vi "subLoadCommandlineArgs.vi"(11 "Options in":T4={"Path"=path "C:/DependencyInspector/src", "Preview?"=FALSE, "Quiet?"=FALSE, "Show help?"=FALSE}) -> (0 "error out":errorcluster, 1 "From command line?":bool, 2 "Item info":T1, 3 "Options":T4={"Path"=path "C:/DependencyInspector/src", "Preview?"=FALSE, "Quiet?"=FALSE, "Show help?"=FALSE})   [LabVIEW 2020, in "SolutionBuilder.lvlib" / "SolutionBuilder.lvclass"]
uses:
  SolutionBuilder.lvclass
  Private/Options.ctl
  Private/FileInfo.ctl
  Private/ProjectInfo.ctl
  Private/ItemInfo.ctl
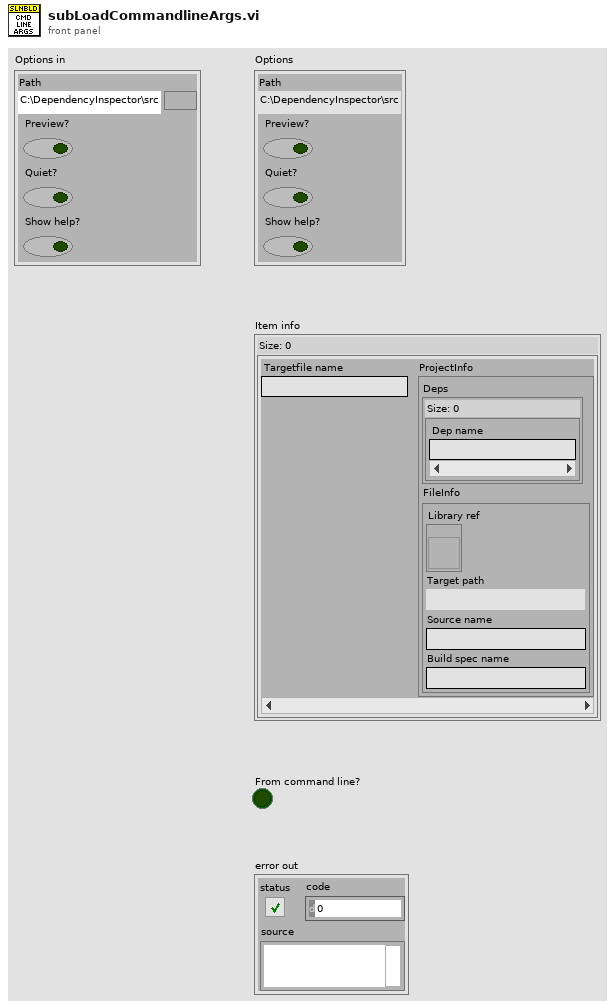
[diagram p1: front panel]
types:
  T1 = typedef "SolutionBuilder.lvlib/SolutionBuilder.lvclass/ItemInfo.ctl" = map{string, T2}
  T2 = typedef "SolutionBuilder.lvlib/SolutionBuilder.lvclass/ProjectInfo.ctl" = cluster{"Deps":set{string}, "FileInfo":T3}
  T3 = typedef "SolutionBuilder.lvlib/SolutionBuilder.lvclass/FileInfo.ctl" = cluster{"Library ref":refnum<vi>, "Target path":path, "Source name":string, "Build spec name":string}
  T4 = typedef "SolutionBuilder.lvlib/SolutionBuilder.lvclass/Options.ctl" = cluster{"Path":path, "Preview?":bool, "Quiet?":bool, "Show help?":bool}
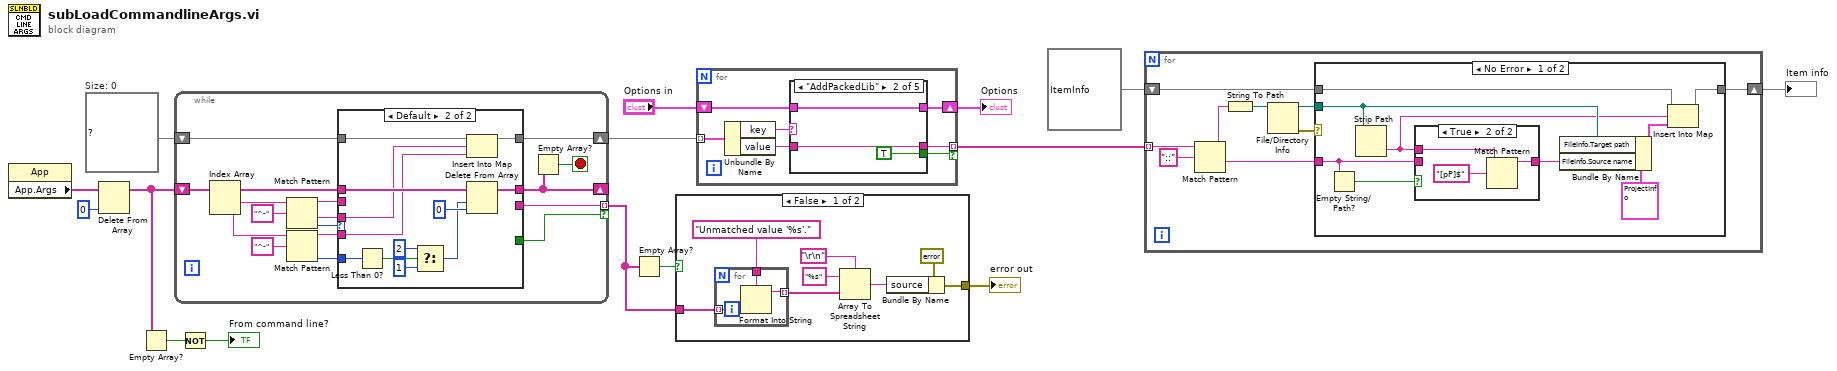
[diagram p0: block diagram]
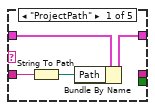
[diagram p3: hidden frame]
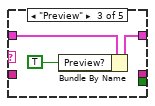
[diagram p4: hidden frame]
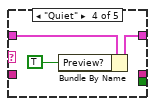
[diagram p5: hidden frame]
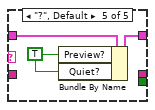
[diagram p6: hidden frame]
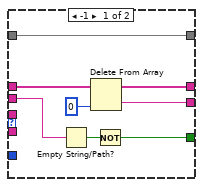
[diagram p7: hidden frame]
diagram:
  w11 = map{string, string} {}  # Size: 0
  n1 = property class="App"() -> ("App.Args"=w7:string[])  [unwired: 2 in, 2 out]
  n2 = Delete From Array(array=w7, index=0) -> (array with subset deleted=w14:string[])  [unwired: 1 in, 1 out]
  n3 = Empty Array?(array=w14) -> (empty?=w13:bool)
  n4 = while {
    shift-right: [w20] -> _
    shift-left: w14 -> [w23]
    shift-right: [w21] -> w8
    shift-left: w11 -> [w22]
    tunnel: [w18] -> w5 mode=indexing if=w17
    stop <- w19 stop-if-true
    n5 = Index Array(array=w23) -> (element #1=w31:string, element #2=w28:string)  [unwired: 2 in]
    n6 = Match Pattern(string=w31, regular expression="^-") -> (before substring=w16:string, after substring=w26:string, offset past match=w27:i32)  [unwired: 1 in, 1 out]
    n7 = Match Pattern(string=w28, regular expression="^-") -> (before substring=w25:string, offset past match=w24:i32)  [unwired: 1 in, 2 out]
    n8 = case shown="Default" w27 {
      tunnel: w26 -> [_ w41]
      tunnel: w25 -> [_ w40]
      tunnel: w24 -> [_ w51]
      tunnel: w23 -> [w38 w49]
      tunnel: [w37 w44] -> w20
      tunnel: w22 -> [w36 w43]
      tunnel: [w36 w42] -> w21
      tunnel: [w35 _] -> w18
      tunnel: [w32 _] -> w17
      tunnel: w16 -> [w34 _]
      frame -1 {
        n9 = Empty String/Path?(string/path=w34) -> (empty?=w33:bool)
        n10 = Delete From Array(array=w38, index=0) -> (deleted portion=w35:string, array with subset deleted=w37:string[])  [unwired: 1 in]
        n11 = Not(x=w33) -> (.not. x?=w32:bool)
      }
      frame Default {
        n12 = Less Than 0?(x=w51) -> (x < 0?=w50:bool)
        n13 = Select(t=2 ("length"), s=w50, f=1 ("length")) -> (s? t:f=w45:i32)
        n14 = Insert Into Map(map in=w43, key=w41, value=w40) -> (map out=w42:map{string, string})  [unwired: 2 out]
        n15 = Delete From Array(array=w49, length=w45, index=0) -> (array with subset deleted=w44:string[])  [unwired: 1 out]
      }
    }
    n16 = Empty Array?(array=w20) -> (empty?=w19:bool)
  }
  n17 = Not(x=w13) -> (.not. x?=→"From command line?":bool)
  n18 = Empty Array?(array=w5) -> (empty?=w4:bool)
  n19 = case shown="False" w4 {
    tunnel: [w58 _] -> w6
    tunnel: w5 -> [w54 _]
    frame False {
      n20 = for {
        tunnel: w54 -> [w62] mode=indexing
        tunnel: [w61] -> w53 mode=indexing
        tunnel: "Unmatched value '%s'." ("format string") -> [w60]
        n21 = Format Into String(format string=w60, w62) -> (resulting string=w61:string)  [unwired: 2 in, 1 out]
      }
      n22 = Array To Spreadsheet String(delimiter (Tab)="\r\n", array=w53, 3:"%s" ("format string")) -> (spreadsheet string=w55:string)
      n23 = Bundle By Name(cluster=errorcluster {"status"=TRUE, "code"=-1, "source"=""} ("error out"), "source"=w55) -> (w58:errorcluster)
    }
    frame True {
    }
  }
  "error out" <- w6
  n24 = for {
    shift-right: [w68] -> w9
    shift-left: "Options in" -> [w69]
    tunnel: w8 -> [w67] mode=indexing
    tunnel: [w64] -> w3 mode=indexing if=w63
    n25 = Unbundle By Name(w67) -> ("key"=w66:string, "value"=w65:string)
    n26 = case shown="\"AddPackedLib\"" w66 {
      tunnel: w69 -> [w73 w76 w79 w82 w85]
      tunnel: w65 -> [w71 w75 _ _ _]
      tunnel: [w72 w76 w78 w81 w84] -> w68
      tunnel: [_ w75 _ _ _] -> w64
      tunnel: [_ TRUE _ _ _] -> w63
      frame "ProjectPath" {
        n27 = String To Path(string=w71) -> (path=w70:path)
        n28 = Bundle By Name(cluster=w73, "Path"=w70) -> (w72:T4)
      }
      frame "AddPackedLib" {
      }
      frame "Preview" {
        n29 = Bundle By Name(cluster=w79, "Preview?"=TRUE) -> (w78:T4)
      }
      frame "Quiet" {
        n30 = Bundle By Name(cluster=w82, "Preview?"=TRUE) -> (w81:T4)
      }
      frame "?", Default {
        w83 = TRUE ("Preview?")
        n31 = Bundle By Name(cluster=w85, "Preview?"=w83, "Quiet?"=w83) -> (w84:T4)
      }
    }
  }
  "Options" <- w9
  n32 = for {
    tunnel: w3 -> [w94] mode=indexing
    shift-right: [w86] -> w1
    shift-left: T1 {} ("Item info") -> [w87]
    n33 = Match Pattern(string=w94, regular expression="::") -> (before substring=w91:string, after substring=w92:string)  [unwired: 1 in, 2 out]
    n34 = String To Path(string=w91) -> (path=w90:path)
    n35 = File/Directory Info(path=w90) -> (path out=w88:path, error out=w89:errorcluster)  [unwired: 1 in, 5 out]
    n36 = case shown="No Error" w89 {
      tunnel: w92 -> [w102 _]
      tunnel: w88 -> [w99 _]
      tunnel: w87 -> [w97 w108]
      tunnel: [w96 w108] -> w86
      frame No Error {
        n37 = Empty String/Path?(string/path=w102) -> (empty?=w103:bool)
        n38 = Strip Path(path=w99) -> (name=w98:string)  [unwired: 1 out]
        n39 = case shown="True" w103 {
          tunnel: w98 -> [_ w106]
          tunnel: [w104 w105] -> w100
          tunnel: w102 -> [w104 _]
          frame False {
          }
          frame True {
            n40 = Match Pattern(string=w106, regular expression="[pP]$") -> (before substring=w105:string)  [unwired: 1 in, 3 out]
          }
        }
        n41 = Bundle By Name(cluster=T2 {"Deps"={}, "FileInfo"={"Library ref"=refnum, "Target path"=path "", "Source name"="", "Build spec name"=""}} ("ProjectInfo"), "FileInfo.Target path"=w99, "FileInfo.Source name"=w100) -> (w95:T2)
        n42 = Insert Into Map(map in=w97, key=w98, value=w95) -> (map out=w96:T1)  [unwired: 2 out]
      }
      frame Error {
      }
    }
  }
  "Item info" <- w1
